vi "Cryotel_logging.vi"() -> ()   [LabVIEW 2019]
uses:
  <vilib>/Analysis/baseanly.llb/Mean (DBL).vi
  <vilib>/Analysis/NI_AALBase.lvlib
panel:
  out "Array 2":i32[](array[numeric])
  out "Error":bool
  out "Error Code":string
  out "ERROR read":string[](array[string])
  in  "Read/new file? 2":bool=TRUE
  out "error out":errorcluster
  in  "Path Cryotel":path=path "C:/RIMAS/logs/Temperature_logs"
  in  "Number of reads":u16=10 min=1 max=50
  in  "EXIT":bool
  in  "Tab Control":enum32{"Page 1", "Page 2"}(tab)
  out "Temperature , Humidity and Pressure":cluster{dbl[], dbl[]}[](graph)
  out "YJ":bool
  out "HK":bool
  out "log file size(s)":i32[](array[numeric])
  out "YJ Heater %":dbl format="%.1f"
  out "HK Heater  %":dbl format="%.1f"
  out "YJ Setpoint (85.0) 2":dbl=85.0 min=-273.0 max=300000.0 step=0.0001 format="%.2f"
  out "HK Setpoint (85.0) 2":dbl=85.0 min=-273.0 max=300000.0 step=0.0001 format="%.2f"
  out "HK Heater Power  (W)":dbl format="%.1f"
  out "YJ Heater (W)":dbl format="%.1f"
  out "Pressure 2":dbl[](array[numeric])
  out "H & T":dbl[](array[numeric])
  out "Time":timestamp[](array[timestamp])
  out "Temperatures-and pressure":dbl[][](array[numeric]) format="%#_8g"
  out "Path 2":path=path "C:/RIMAS_logs/Temperature_pressure_logs/Temperature_log"
  in  "error in (no error) 4":errorcluster
  in  "Read/new file?":bool=TRUE
  in  "Reading Interval (sec)":dbl=5.0 min=0.2 max=10.0 step=0.0001 format="%.1f"
  out "Data":sgl[](array[numeric])
  out "Array":string[](array[string])
  out "read string array":string[](array[string])
  in  "?":string
  in  "Command":u16(ring) items=["STATUS", "COOLER", "E", "ERROR", "KD", "KI", "KP", "LOGIN", "LOGOUT", "MODE", "P", "PWOUT", "SENSOR", "TC", "TEMP RJ", "TTARGET", "VERSION"]
  in  "VISA Resource (write)":refnum<visa-resource-name>="COM17"
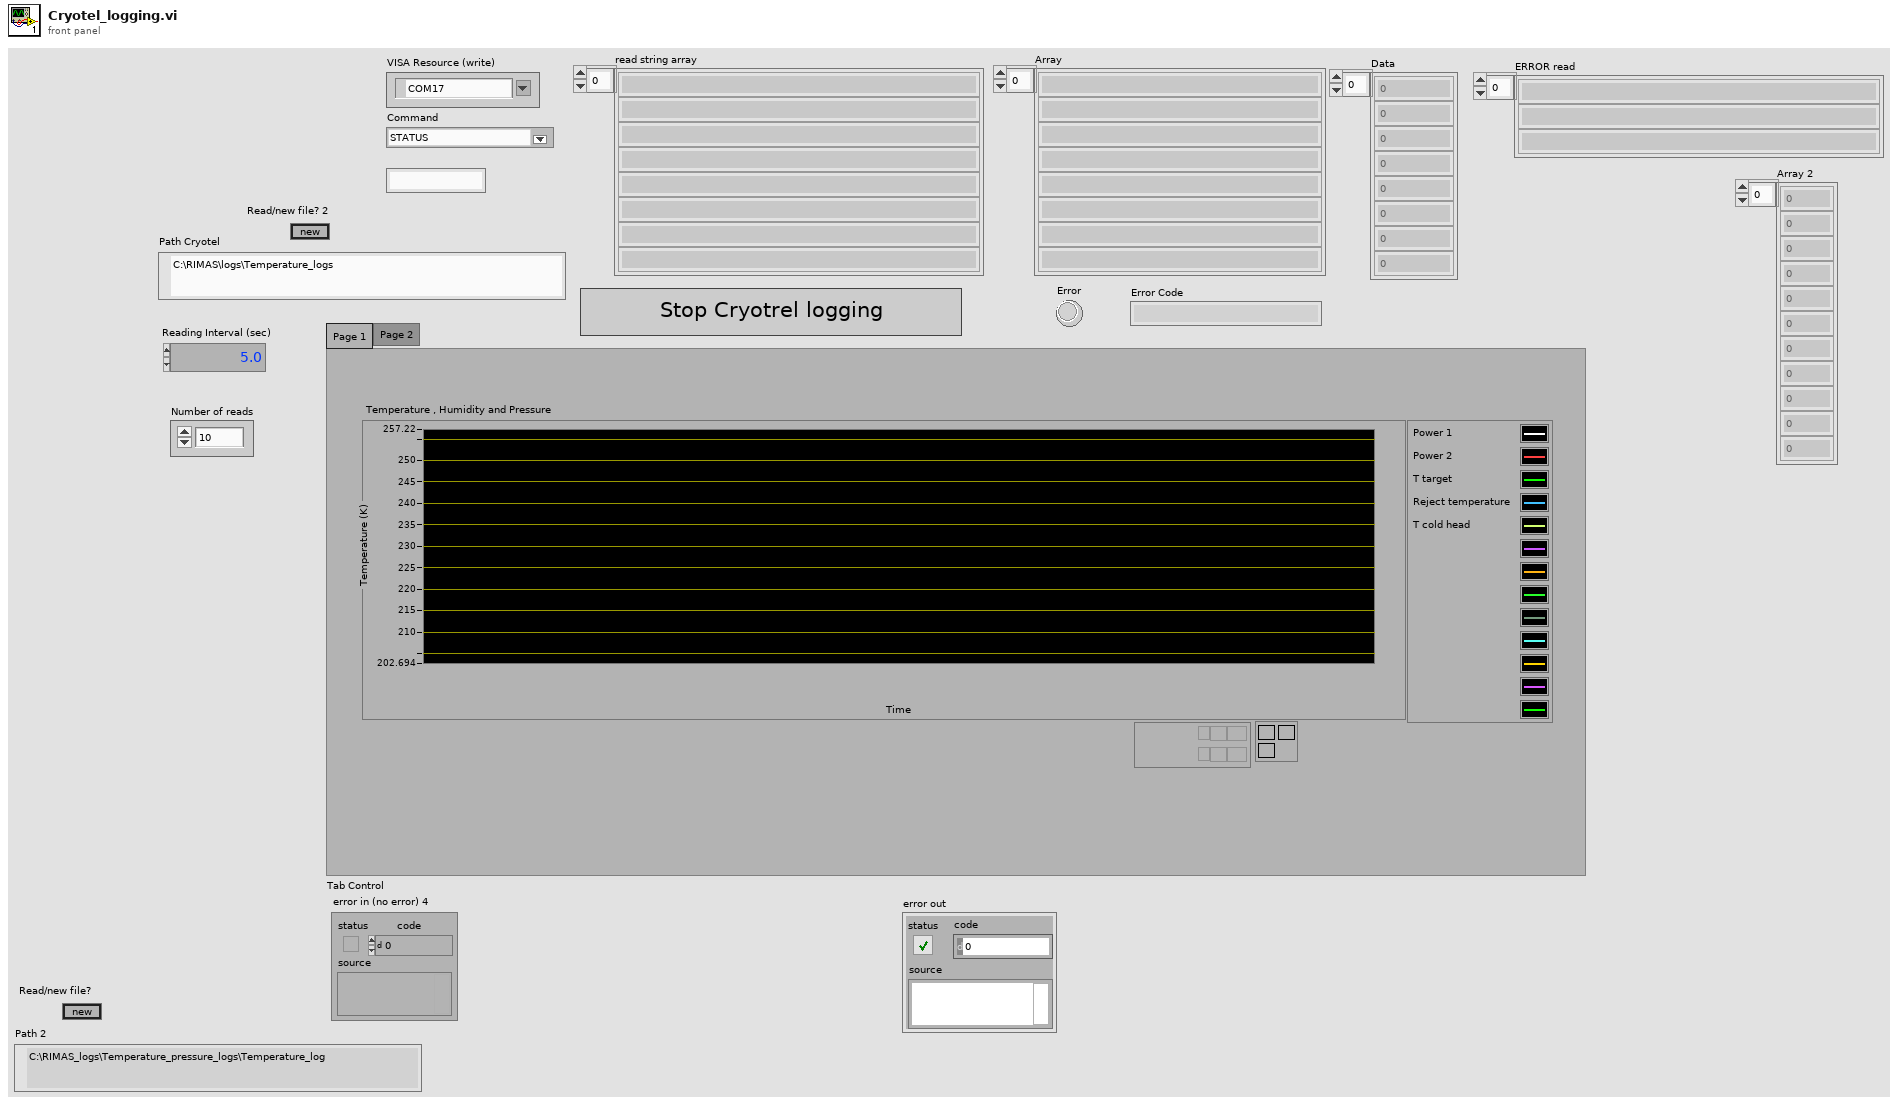
[diagram p1: front panel]
types:
  T1 = enum8{"Enabled", "Disabled", "Disabled and Grayed Out"}
  T2 = enum16{"open", "replace", "create", "open or create", "replace or create", "replace or create with confirmation"}
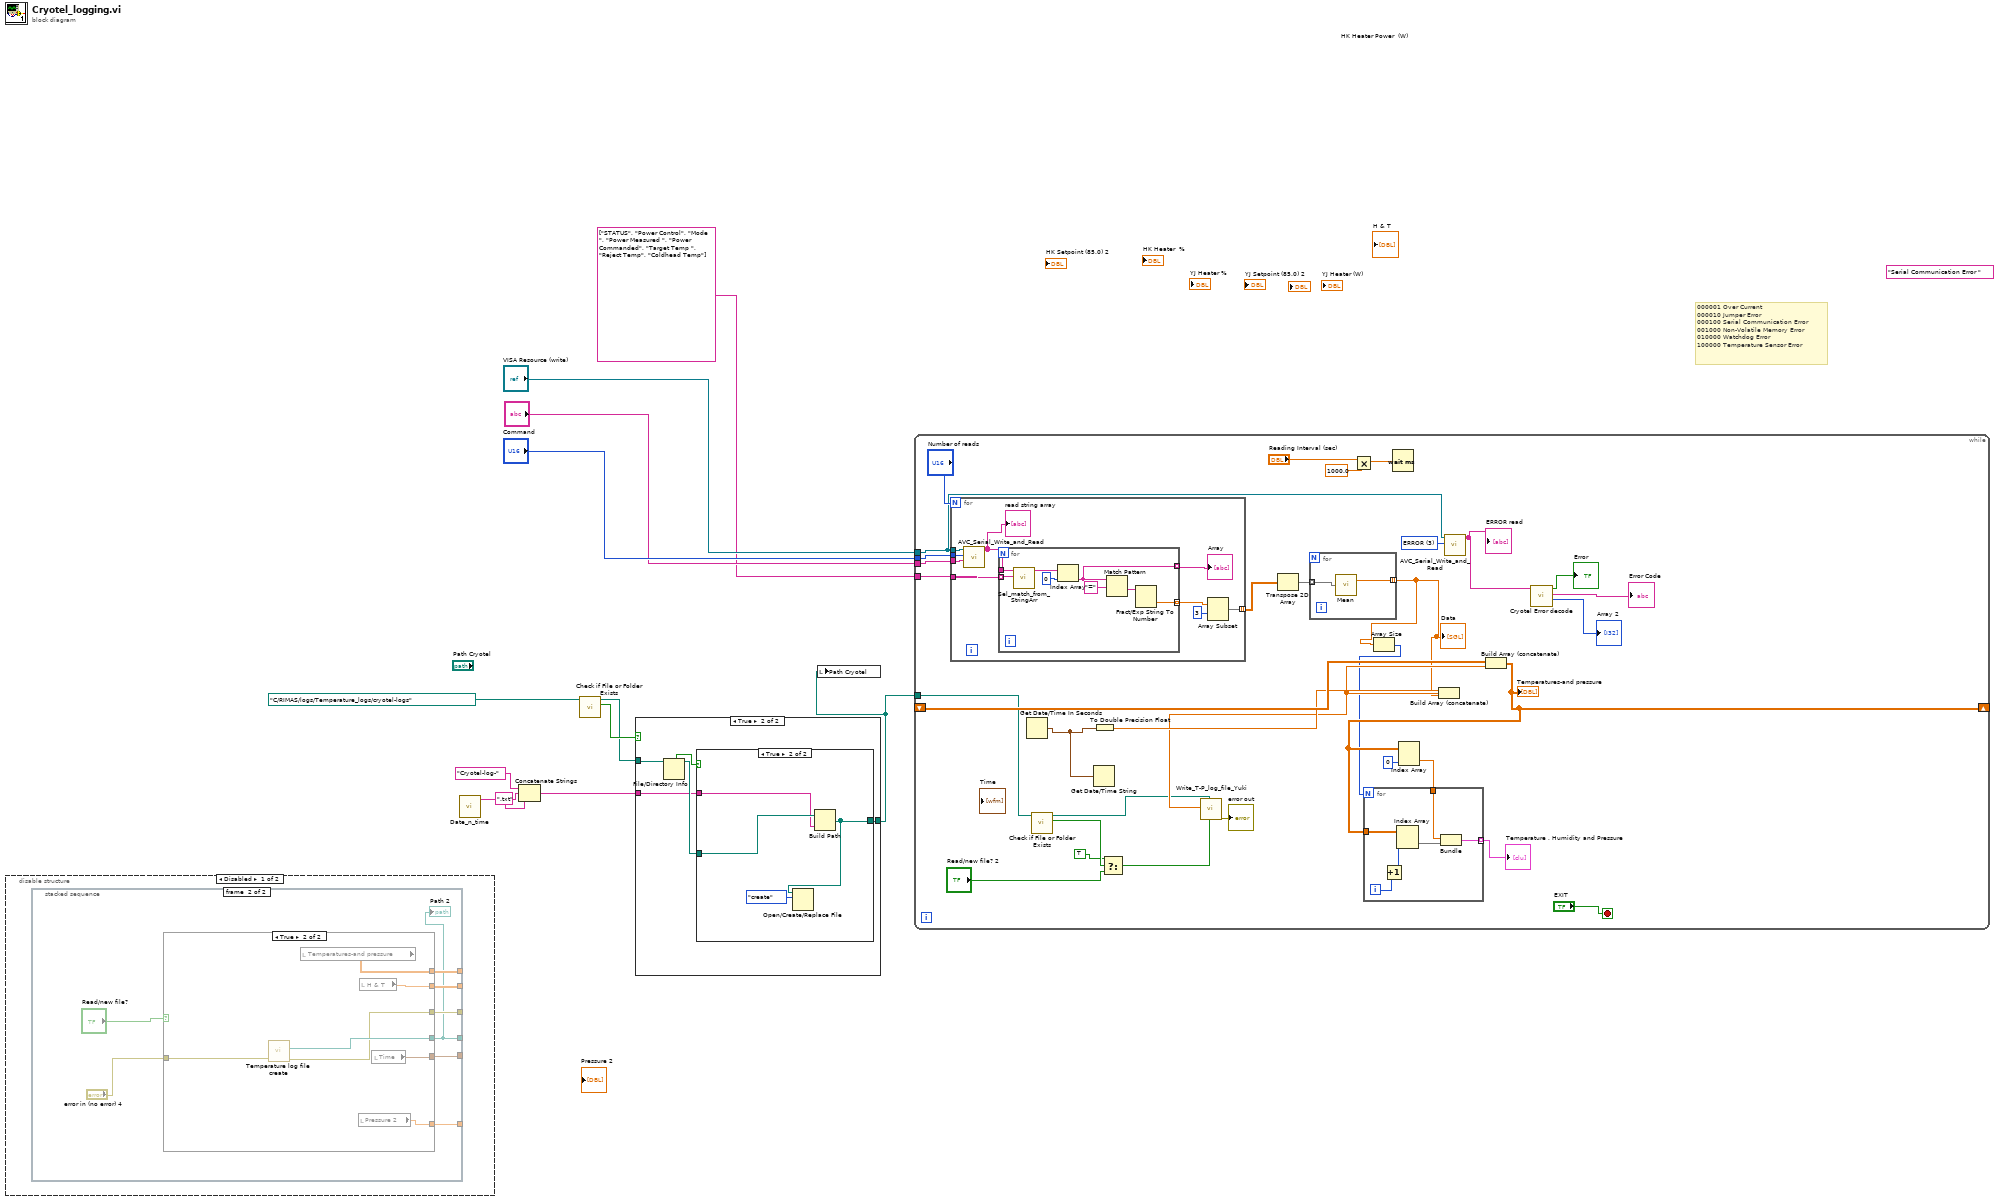
[diagram p0: block diagram]
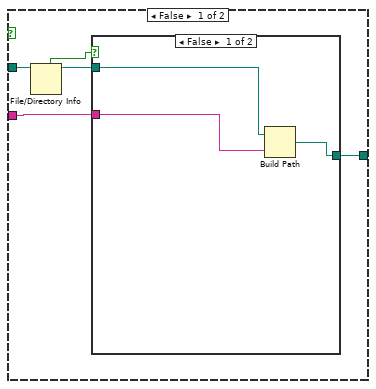
[diagram p2: hidden frame]
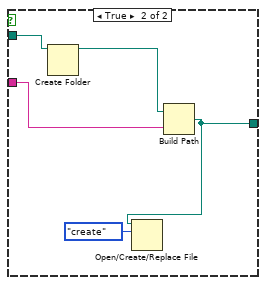
[diagram p3: hidden frame]
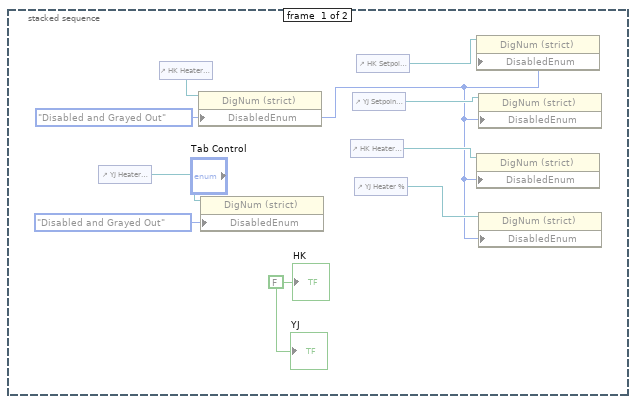
[diagram p5: hidden frame]
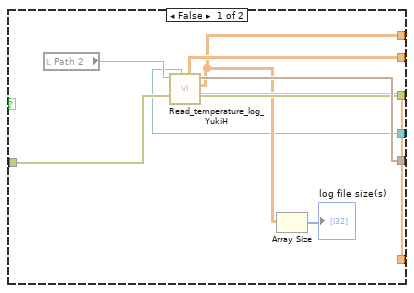
[diagram p6: hidden frame]
diagram:
  (unwired) "Serial Communication Error "
  # "000001 Over Current \n000010 Jumper Error \n000100 Serial Communication Error \n001000 Non-Volatile Memory Error \n010000 Watchdog Error \n100000 Temperature Sensor Error"
  n1 = disable-structure shown="Disabled" {
    frame Disabled {
      n2 = stacked-sequence {
        tunnel: [_ w29] -> _
        tunnel: [_ w26] -> _
        tunnel: [_ w25] -> _
        tunnel: [_ w24] -> _
        tunnel: [_ w23] -> _
        tunnel: [_ w22] -> _
        frame #0 {
          w18 = FALSE ("HK")
          w13 = T1."Disabled and Grayed Out" ("Disabled")
          n3 = control-ref of="YJ Heater (W)"() -> (w21:refnum<vi>)
          n4 = control-ref of="HK Heater Power  (W)"() -> (w20:refnum<vi>)
          n5 = property class="DigNum (strict)"(reference=w20, "DisabledEnum"=w13) -> ()  [unwired: 1 in, 2 out]
          n6 = property class="DigNum (strict)"(reference=w21, "DisabledEnum"=T1."Disabled and Grayed Out" ("Disabled")) -> ()  [unwired: 1 in, 2 out]
          n7 = control-ref of="HK Heater  %"() -> (w15:refnum<vi>)
          n8 = control-ref of="YJ Setpoint (85.0) 2"() -> (w16:refnum<vi>)
          n9 = control-ref of="YJ Heater %"() -> (w14:refnum<vi>)
          n10 = control-ref of="HK Setpoint (85.0) 2"() -> (w17:refnum<vi>)
          n11 = property class="DigNum (strict)"(reference=w17, "DisabledEnum"=w13) -> ()  [unwired: 1 in, 2 out]
          n12 = property class="DigNum (strict)"(reference=w15, "DisabledEnum"=w13) -> ()  [unwired: 1 in, 2 out]
          n13 = property class="DigNum (strict)"(reference=w16, "DisabledEnum"=w13) -> ()  [unwired: 1 in, 2 out]
          n14 = property class="DigNum (strict)"(reference=w14, "DisabledEnum"=w13) -> ()  [unwired: 1 in, 2 out]
          "HK" <- w18
          "YJ" <- w18
        }
        frame #1 {
          n15 = case shown="True" "Read/new file?" {
            tunnel: [w36 w38] -> w29
            tunnel: "error in (no error) 4" -> [w36 w44]
            tunnel: [w32 w43] -> w26
            tunnel: [w37 w42] -> w25
            tunnel: [w33 w40] -> w24
            tunnel: [w34 w41] -> w23
            tunnel: [w30 w39] -> w22
            frame False {
              n16 = local read "Path 2"() -> (w31:path)
              n17 = call "Read_temperature_log_YukiH.vi"("Log File path"=w31) -> ("Pressure"=w33:dbl[], "temperature"=w32:dbl[][], "time stamp"=w37:timestamp[], "H&T"=w34:dbl[][], "Log file name"=w30:path)  [unwired: 6 in]
              n18 = Array Size(array=w32) -> (size(s)=→"log file size(s)":i32[])
            }
            frame True {
              n19 = call "Temperature log file create.vi"("error in (no error)"=w44) -> ("error in (no error)"=w38:errorcluster, "Temperature log file"=w39:path)  [unwired: 8 in, 1 out]
              n20 = local read "Temperatures-and pressure"() -> (w43:dbl[][])
              n21 = local read "Pressure 2"() -> (w40:dbl[])
              n22 = local read "H & T"() -> (w41:dbl[])
              n23 = local read "Time"() -> (w42:timestamp[])
            }
          }
          "Path 2" <- w22
        }
      }
    }
    frame Enabled {
    }
  }
  n24 = call <userlib>:"Date_n_time.vi"() -> ("date string"=w5:string)  [unwired: 9 in, 2 out]
  n25 = Concatenate Strings("Cryotel-log-", w5, ".txt" ("string")) -> (w2:string)
  n26 = call <vilib>:"Check if File or Folder Exists.vi"("path"=path "C:/RIMAS/logs/Temperature_logs/cryotel-logs" ("Path Cryotel")) -> ("file or folder exists?"=w8:bool, "dup path"=w7:path)  [unwired: 8 in, 1 out]
  n27 = case shown="True" w8 {
    tunnel: w7 -> [w49 w62]
    tunnel: [w45 w59] -> w1
    tunnel: w2 -> [w46 w58]
    frame False {
      n28 = File/Directory Info(path=w49) -> (path out=w47:path, directory=w48:bool)  [unwired: 1 in, 5 out]
      n29 = case shown="False" w48 {
        tunnel: w47 -> [w52 w57]
        tunnel: w46 -> [w51 w55]
        tunnel: [w50 w53] -> w45
        frame False {
          n30 = Build Path(base path=w52, name or relative path=w51) -> (appended path=w50:path)
        }
        frame True {
          n31 = Create Folder(path (use dialog)=w57) -> (created path=w56:path)  [unwired: 2 in, 2 out]
          n32 = Build Path(base path=w56, name or relative path=w55) -> (appended path=w53:path)
          n33 = Open/Create/Replace File(file path (use dialog)=w53, operation (0:open)=T2."create") -> ()  [unwired: 4 in, 3 out]
        }
      }
    }
    frame True {
      n34 = File/Directory Info(path=w62) -> (path out=w60:path, directory=w61:bool)  [unwired: 1 in, 5 out]
      n35 = case shown="True" w61 {
        tunnel: w60 -> [w63 w67]
        tunnel: [w63 w65] -> w59
        tunnel: w58 -> [_ w64]
        frame False {
        }
        frame True {
          n36 = Build Path(base path=w67, name or relative path=w64) -> (appended path=w65:path)
          n37 = Open/Create/Replace File(file path (use dialog)=w65, operation (0:open)=T2."create") -> ()  [unwired: 4 in, 3 out]
        }
      }
    }
  }
  n38 = local write "Path Cryotel"(w1) -> ()
  n39 = while {
    tunnel: "VISA Resource (write)" -> [w73]
    tunnel: "Command" -> [w87]
    tunnel: "?" -> [w88]
    tunnel: string[] ["STATUS", "Power Control", "Mode  ", "Power Measured ", "Power Commanded", "Target Temp ", "Reject Temp", "Coldhead Temp"] -> [w100]
    shift-right: [w91] -> _
    shift-left: _ -> [w99]
    tunnel: w1 -> [w79]
    stop <- "EXIT" stop-if-true
    w72 = u16 3 items=["STATUS", "COOLER", "E", "ERROR", "KD", "KI", "KP", "LOGIN", "LOGOUT", "MODE", "P", "PWOUT", "SENSOR", "TC", "TEMP RJ", "TTARGET", "VERSION"] ("Command")
    n40 = for {
      N: "Number of reads" -> [_]
      tunnel: w100 -> [w117]
      tunnel: w88 -> [w115]
      tunnel: w87 -> [w114]
      tunnel: w73 -> [w113]
      tunnel: [w110] -> w86 mode=indexing
      n41 = call "AVC_Serial_Write_and_Read.vi"("Command Options"=w115, "Command"=w114, "VISA Resource (write)"=w113) -> ("read string array"=w109:string[])  [unwired: 8 in]
      "read string array" <- w109
      n42 = for {
        tunnel: w117 -> [w122] mode=indexing
        tunnel: w109 -> [w125]
        tunnel: [w120] -> w116 mode=indexing
        tunnel: [w121] -> w111 mode=indexing
        n43 = call <userlib>:"Sel_match_from_StringArr.vi"("String to match"=w122, "String Array In"=w125) -> ("String Array Matched"=w124:string[])  [unwired: 5 in, 4 out]
        n44 = Index Array(array=w124, index=0) -> (element=w120:string)
        n45 = Match Pattern(string=w120, regular expression="=") -> (after substring=w118:string)  [unwired: 1 in, 3 out]
        n46 = Fract/Exp String To Number(string=w118) -> (number=w121:dbl)  [unwired: 3 in, 1 out]
      }
      "Array" <- w116
      n47 = Array Subset(array=w111, index=3) -> (w110:dbl[])  [unwired: 1 in]
    }
    n48 = Get Date/Time In Seconds() -> (seconds since 1Jan1904=w94:timestamp)
    n49 = call <vilib>:"Check if File or Folder Exists.vi"("path"=w79) -> ("file or folder exists?"=w78:bool, "dup path"=w74:path)  [unwired: 8 in, 1 out]
    n50 = Get Date/Time String(seconds (now)=w94) -> ()  [unwired: 2 in, 2 out]
    n51 = To Double Precision Float(number=w94) -> (double precision float=w93:dbl)
    n52 = Select(t=TRUE, s=w78, f="Read/new file? 2") -> (s? t:f=w75:bool)
    n53 = Transpose 2D Array(2D array=w86) -> (transposed array=w85:dbl[][])
    n54 = for {
      tunnel: w85 -> [w108] mode=indexing
      tunnel: [w107] -> w82 mode=indexing
      n55 = call-poly <vilib>:"Mean.vi"("X"=w108) -> ("mean"=w107:dbl)  [unwired: 1 out]
    }
    "Data" <- w82
    n56 = Multiply(x="Reading Interval (sec)", y=1000.0) -> (x*y=w96:dbl)
    n57 = Array Size(array=w82) -> (size(s)=w81:i32)
    n58 = Wait (ms)(milliseconds to wait=w96) -> ()  [unwired: 1 out]
    n59 = Build Array (concatenate)(w93, w82) -> (w84:dbl[])
    n60 = call "Write_T-P_log_file_Yuki.vi"("append to file? (new file:F)"=w75, "Log file path (dialog if empty)"=w74, "Array in"=w84) -> ("error out"=→"error out":errorcluster)  [unwired: 6 in, 2 out]
    n61 = call "AVC_Serial_Write_and_Read.vi"("Command"=w72, "VISA Resource (write)"=w73) -> ("read string array"=w71:string[])  [unwired: 9 in]
    "ERROR read" <- w71
    n62 = Build Array (concatenate)(w99, w84) -> (w91:dbl[][])
    "Temperatures-and pressure" <- w91
    n63 = Index Array(array=w91, index (col)=0 ("disabled index (col)")) -> (element=w90:dbl[])  [unwired: 1 in]
    n64 = for {
      N: w81 -> [_]
      tunnel: w91 -> [w106]
      tunnel: w90 -> [w105]
      tunnel: [w103] -> w80 mode=indexing
      i -> [w102]
      n65 = Increment(x=w102) -> (x+1=w101:i32)
      n66 = Index Array(array=w106, index (col)=w101) -> (element=w104:dbl[])  [unwired: 1 in]
      n67 = Bundle(w105, w104) -> (w103:cluster{dbl[], dbl[]})  [unwired: 1 in]
    }
    "Temperature , Humidity and Pressure" <- w80
    n68 = call <userlib>:"Cryotel Error decode.vi"("read string array"=w71) -> ("Array 2"=→"Array 2":i32[], "Error Code"=→"Error Code":string, "Error"=→"Error":bool)  [unwired: 8 in]
  }
